vi "Pod setpoints Optimization latency test.vi"() -> ()   [LabVIEW 2020]
uses:
  <vilib>/Analysis/coordinate.llb/Angle Units.ctl
  <vilib>/Analysis/coordinate.llb/Angle Range (Degree).ctl
  <vilib>/numeric/Random Number (Range) DBL.vi
  <vilib>/Analysis/coordinate.llb/Wrap Angle (scalar).vi
  <vilib>/Analysis/NI_AAL_Angle.lvlib
panel:
  out "Max Setpoint Diff":dbl
  out "Current Pod Steering (deg)":cluster{"LF":dbl, "LB":dbl, "RF":dbl, "RB":dbl}
  out "Angle Setpoint":dbl[](array[numeric])
  out "Counter":dbl
  out "New Pod Steering":T1
  in  "Max Turn":dbl
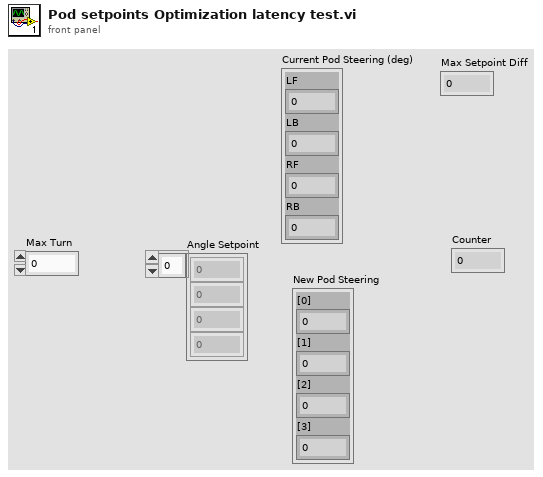
[diagram p1: front panel]
types:
  T1 = cluster{"[0]":dbl, "[1]":dbl, "[2]":dbl, "[3]":dbl}
  T2 = cluster{"LF":dbl[], "LB":dbl[], "RF":dbl[], "RB":dbl[]}
  T3 = cluster{"number":dbl, "number":dbl, "number":dbl}
  T4 = typedef "Pod Setpoints.ctl" = cluster{"Left Front":cluster{"Velocity":dbl, "Theta":dbl}, "Left Back":cluster{"Velocity":dbl, "Theta":dbl}, "Right Front":cluster{"Velocity":dbl, "Theta":dbl}, "Right Back":cluster{"Velocity":dbl, "Theta":dbl}}
  T5 = typedef "NI_AAL_Angle.lvlib/Angle Units.ctl" = i32
  T6 = typedef "NI_AAL_Angle.lvlib/Angle Range (Degree).ctl" = u16
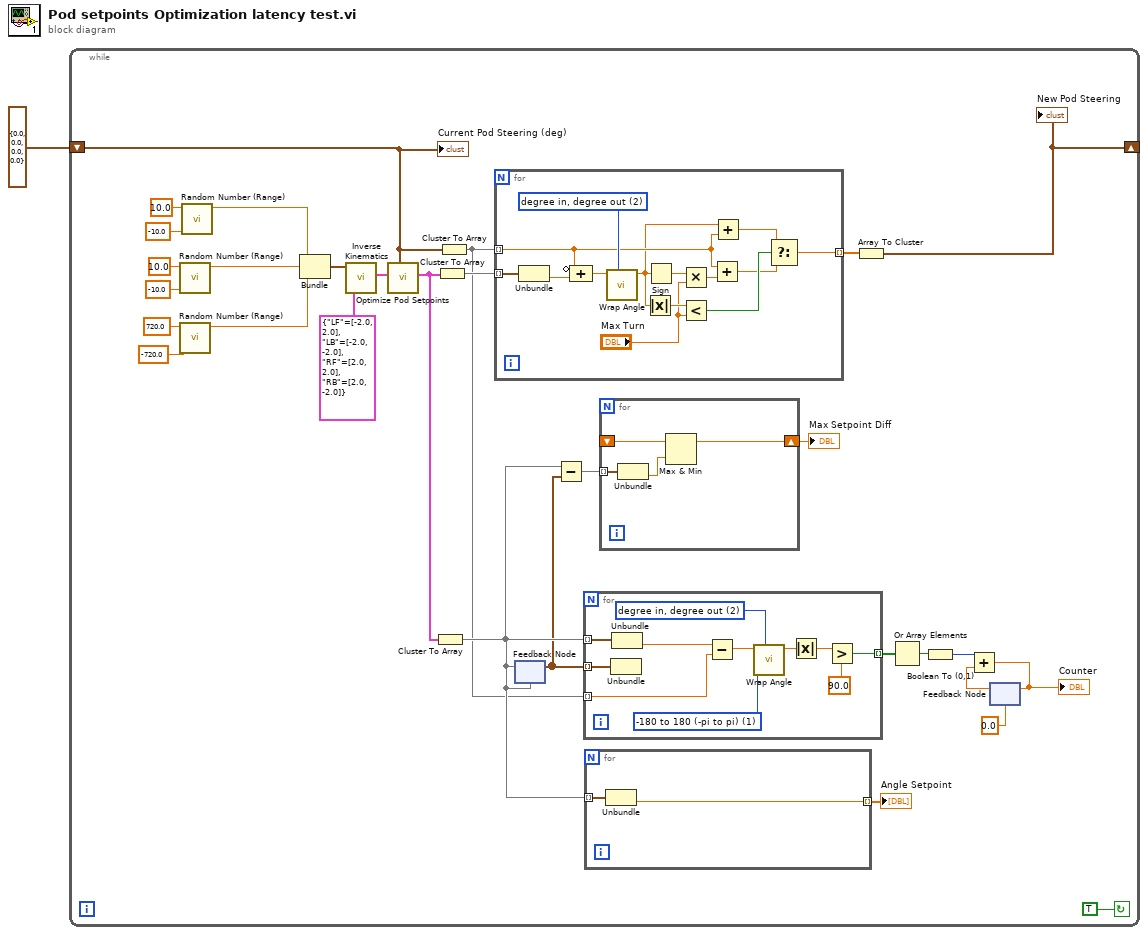
[diagram p0: block diagram]
diagram:
  n1 = while {
    shift-right: [w16] -> _
    shift-left: cluster{"LF":dbl, "LB":dbl, "RF":dbl, "RB":dbl} {"LF"=0.0, "LB"=0.0, "RF"=0.0, "RB"=0.0} ("Current Pod Steering (deg)") -> [w17]
    stop <- TRUE continue-if-true
    n2 = call-poly <vilib>:"Random Number (Range).vi"("lower bound (0)"=-10.0, "upper bound (100)"=10.0) -> ("number"=w22:dbl)  [unwired: 9 in]
    n3 = call-poly <vilib>:"Random Number (Range).vi"("lower bound (0)"=-720.0, "upper bound (100)"=720.0) -> ("number"=w21:dbl)  [unwired: 9 in]
    n4 = call-poly <vilib>:"Random Number (Range).vi"("lower bound (0)"=-10.0, "upper bound (100)"=10.0) -> ("number"=w23:dbl)  [unwired: 9 in]
    n5 = Bundle("number"=w23, "number"=w22, "number"=w21) -> (w29:T3)  [unwired: 1 in]
    n6 = call "Inverse Kinematics.vi"("Radii (ft)"=T2 {"LF"=[-2.0, 2.0], "LB"=[-2.0, -2.0], "RF"=[2.0, 2.0], "RB"=[2.0, -2.0]} ("Radii"), "Target Velocity (ft/s and deg/s)"=w29) -> ("Pod Setpoints (ft/s and deg)"=w31:T4)  [unwired: 7 in, 2 out]
    n7 = call "Optimize Pod Setpoints.vi"("Current Pod Steering (deg)"=w17, "Initial Pod Setpoints (ft/s and deg)"=w31) -> ("Optimized Pod Setpoints (ft/s and deg)"=w8:T4)  [unwired: 9 in]
    n8 = Cluster To Array(cluster=w8) -> (array=w6:cluster{"Velocity":dbl, "Theta":dbl}[])
    n9 = Cluster To Array(cluster=w8) -> (array=w19:cluster{"Velocity":dbl, "Theta":dbl}[])
    n10 = Cluster To Array(cluster=w17) -> (array=w4:dbl[])
    n11 = for {
      tunnel: w19 -> [w62] mode=indexing
      tunnel: w4 -> [w54] mode=indexing
      tunnel: [w49] -> w18 mode=indexing
      w59 = T5 2 items=["radian in, radian out", "radian in, degree out", "degree in, degree out", "degree in, radian out"] ("angle units")
      n12 = Unbundle(w62) -> ("Theta"=w61:dbl)  [unwired: 1 out]
      n13 = Compound Arithmetic op=ADD(invert w54, w61) -> (w60:dbl)
      n14 = call-poly <vilib>:"Wrap Angle.vi"("angle units"=w59, "angle in"=w60) -> ("angle out"=w53:dbl)  [unwired: 8 in, 1 out]
      n15 = Absolute Value(x=w53) -> (abs(x)=w58:dbl)
      n16 = Sign(1:w53) -> (0:w57:dbl)
      n17 = Multiply(x=w57, y="Max Turn") -> (x*y=w55:dbl)
      n18 = Less?(x=w58, y="Max Turn") -> (x < y?=w52:bool)
      n19 = Add(x=w54, y=w55) -> (x+y=w50:dbl)
      n20 = Add(x=w53, y=w54) -> (x+y=w51:dbl)
      n21 = Select(t=w51, s=w52, f=w50) -> (s? t:f=w49:dbl)
    }
    n22 = feedback #1(w6) -> (w5:cluster{"Velocity":dbl, "Theta":dbl}[])
    n23 = feedback-in #1(w6) -> ()
    n24 = Subtract(x=w6, y=w5) -> (x-y=w3:cluster{"Velocity":dbl, "Theta":dbl}[])
    n25 = for {
      tunnel: w6 -> [w48] mode=indexing
      tunnel: [w40] -> w14 mode=indexing
      tunnel: w5 -> [w39] mode=indexing
      tunnel: w4 -> [w38] mode=indexing
      w44 = T5 2 items=["radian in, radian out", "radian in, degree out", "degree in, degree out", "degree in, radian out"] ("angle units")
      w45 = T6 1 items=["none", "-180 to 180 (-pi to pi)", "0 to 360 (0 to 2pi)"] ("angle range")
      n26 = Unbundle(w39) -> ()  [unwired: 2 out]
      n27 = Unbundle(w48) -> ("Theta"=w47:dbl)  [unwired: 1 out]
      n28 = Subtract(x=w47, y=w38) -> (x-y=w46:dbl)
      n29 = call-poly <vilib>:"Wrap Angle.vi"("angle units"=w44, "angle range"=w45, "angle in"=w46) -> ("angle out"=w43:dbl)  [unwired: 7 in, 1 out]
      n30 = Absolute Value(x=w43) -> (abs(x)=w42:dbl)
      n31 = Greater?(x=w42, y=90.0) -> (0:w40:bool)
    }
    n32 = for {
      tunnel: w6 -> [w37] mode=indexing
      tunnel: [w36] -> w7 mode=indexing
      n33 = Unbundle(w37) -> ("Theta"=w36:dbl)  [unwired: 1 out]
    }
    "Angle Setpoint" <- w7
    n34 = for {
      tunnel: w3 -> [w35] mode=indexing
      shift-right: [w33] -> w2
      shift-left: _ -> [w32]
      n35 = Unbundle(w35) -> ("Theta"=w34:dbl)  [unwired: 1 out]
      n36 = Max & Min(x=w32, y=w34) -> (max(x,y)=w33:dbl)  [unwired: 1 out]
    }
    "Max Setpoint Diff" <- w2
    n37 = Array To Cluster(array=w18) -> (cluster=w16:T1)
    "New Pod Steering" <- w16
    n38 = Or Array Elements(Boolean array=w14) -> (logical OR=w13:bool)
    n39 = Boolean To (0,1)(Boolean=w13) -> (0, 1=w11:i16)
    n40 = feedback #2(0.0) -> (w10:dbl)
    n41 = Add(x=w11, y=w10) -> (x+y=w9:dbl)
    "Counter" <- w9
    n42 = feedback-in #2(w9) -> ()
    "Current Pod Steering (deg)" <- w17
  }
